vi "PC_read_FIFO_Health_and_CPU_and_memory.vi"(8 "error in (no error)":errorcluster) -> (0 "error out":errorcluster, 2 "Cluster":T2, 3 "output cluster":T1)   [LabVIEW 2020]
uses:
  RT_only_FIFO_Health.ctl
  RT_CPU_load.ctl
  RT_FIFO_Health.ctl
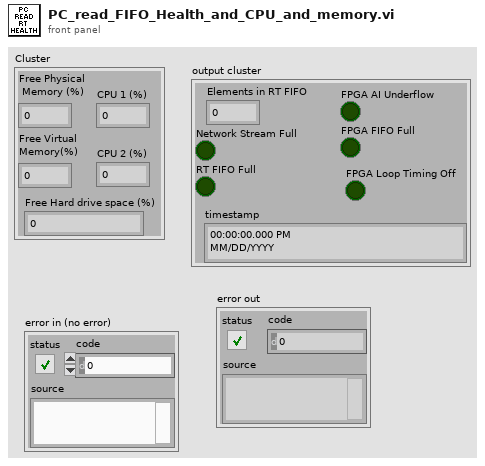
[diagram p1: front panel]
types:
  T1 = typedef "RT_only_FIFO_Health.ctl" = cluster{"Elements in RT FIFO":i32, "Network Stream Full":bool, "RT FIFO Full":bool, "FPGA AI Underflow":bool, "FPGA FIFO Full":bool, "FPGA Loop Timing Off":bool, "timestamp":timestamp}
  T2 = cluster{"CPU 1 (%)":dbl, "CPU 2 (%)":dbl, "Free Physical\n Memory (%)":dbl, "Free Virtual\nMemory(%)":dbl, "Free Hard drive space (%)":dbl}
  T3 = typedef "RT_CPU_load.ctl" = cluster{"Total (%)":dbl, "Time Critical (%)":dbl, "Timed Structures (%)":dbl, "High (%)":dbl, "Above Normal (%)":dbl, "Normal (%)":dbl, "Background (%)":dbl, "Idle (%)":dbl, "ISR (%)":dbl, "ISR (%) 2":dbl, "Idle (%) 2":dbl, "Background (%) 2":dbl, "Normal (%) 2":dbl, "Above Normal (%) 2":dbl, "High (%) 2":dbl, "Timed Structures (%) 2":dbl, "Time Critical (%) 2":dbl, "Total (%) 2":dbl}
  T4 = typedef "RT_FIFO_Health.ctl" = cluster{dbl, dbl, dbl, "TotalPhysMem":dbl, "FreePhysMem":dbl, "TotalVirtMem":dbl, "FreeVirtMem":dbl, "TotalDisk":dbl, "FreeDisk":dbl}
  T5 = cluster{"Total (%)":dbl, "Total (%) 2":dbl, dbl, dbl, dbl}
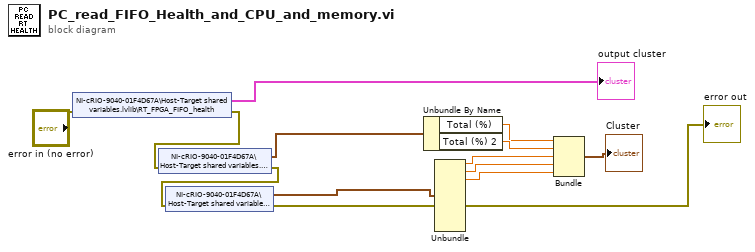
[diagram p0: block diagram]
diagram:
  n1 = shared-variable "NI-cRIO-9040-01F4D67A\\Host-Target shared variables.lvlib\\RT_FPGA_FIFO_health"(error in="error in (no error)") -> (→"output cluster":T1, error out=w2:errorcluster)
  n2 = shared-variable "NI-cRIO-9040-01F4D67A\\Host-Target shared variables.lvlib\\RT CPU Load"(error in=w2) -> (w6:T3, error out=w3:errorcluster)
  n3 = shared-variable "NI-cRIO-9040-01F4D67A\\Host-Target shared variables.lvlib\\RT_Memory"(error in=w3) -> (w7:T4, error out=→"error out":errorcluster)
  n4 = Unbundle By Name(w6) -> ("Total (%)"=w8:dbl, "Total (%) 2"=w9:dbl)
  n5 = Unbundle(w7) -> (w10:dbl, w11:dbl, w12:dbl)  [unwired: 6 out]
  n6 = Bundle("Total (%)"=w8, "Total (%) 2"=w9, w10, w11, w12) -> (→"Cluster":T5)  [unwired: 1 in]
